vi "Initialize 1553 Module.vi"(4 "Debug Flags (0x3000 0000)":T2, 6 "self test mode (none)":T4(ring), 8 "error in":errorcluster, 10 "BIU number (0)":u8, 11 "module number (0)":u32) -> (0 "error out":errorcluster {"code" format="%x"}, 3 "module reference":T1)   [LabVIEW 2020, in "AIM MIL-STD-1553 Hardware API.lvlib"]
uses:
  AIM MIL-STD-1553 Hardware API.lvlib
  Module Reference.ctl
  <instrlib>/_AIM MIL-STD-1553/PCI-1553 Mid-Level Release/1553 Utility - RT Mode Global.vi
panel:
  out "Reset Information":T3 {"Sim Buffer Addr" format="%08x"; "Sim Buffer Size" format="%08x"; "Bus Mon Buffer Addr" format="%08x"; "Bus Mon Buffer Size" format="%08x"}
  # "Simulator Buffer"
  # "Size"
  # "Address"
  # "Bus Monitor Buffer"
  # "Size"
  # "Address"
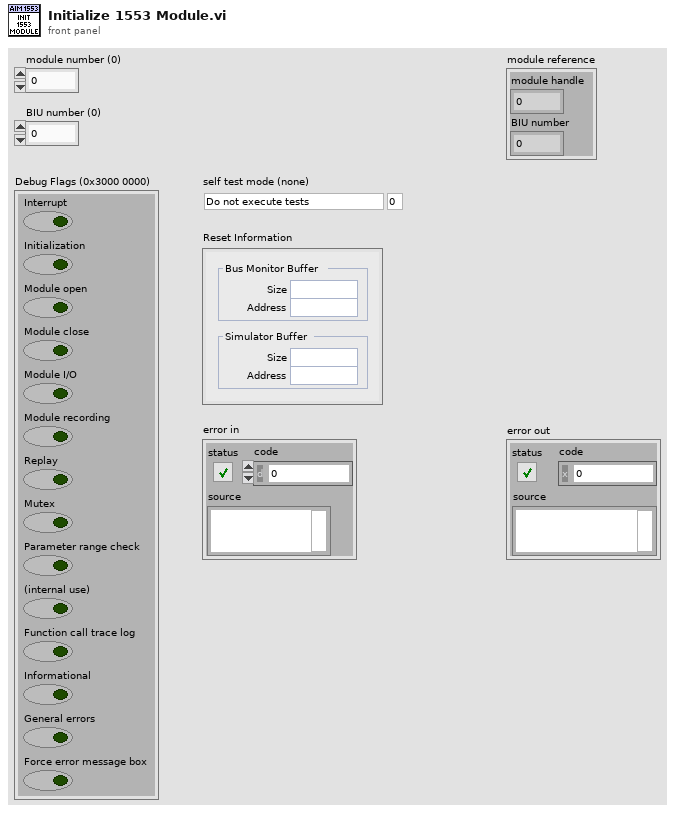
[diagram p1: front panel]
types:
  T1 = typedef "AIM MIL-STD-1553 Hardware API.lvlib/Module Reference.ctl" = cluster{"module handle":u32, "BIU number":u8}
  T2 = cluster{"Interrupt":bool, "Initialization":bool, "Module open":bool, "Module close":bool, "Module I/O":bool, "Module recording":bool, "Replay":bool, "Mutex":bool, "Parameter range check":bool, "(internal use)":bool, "Function call trace log":bool, "Informational":bool, "General errors":bool, "Force error message box":bool}
  T3 = cluster{"Bus Mon Buffer Size":u8, "Sim Buffer Size":u8, "Bus Mon Buffer Addr":u32, "Sim Buffer Addr":u32}
  T4 = enum16{"Do not execute tests", "Execute all tests", "Board enable test", "Internal self-test", "Global RAM test for BIU control block", "Global RAM test for BIU BC/RT descriptor", "Global RAM test for BIU bus monitor", "Shared RAM test from 0x100000", "Shared RAM test for CMD area", "Shared RAM test for ACK area", "Transfer test", "Interrupt test", "DAC test for bus A", "DAC test for bus B", "Timing test"}
  T5 = enum16{"Execute all tests", "Board enable test", "Internal self-test", "Global RAM test for BIU control block", "Global RAM test for BIU BC/RT descriptor", "Global RAM test for BIU bus monitor", "Shared RAM test from 0x100000", "Shared RAM test for CMD area", "Shared RAM test for ACK area", "Transfer test", "Interrupt test", "DAC test for bus A", "DAC test for bus B", "Timing test"}
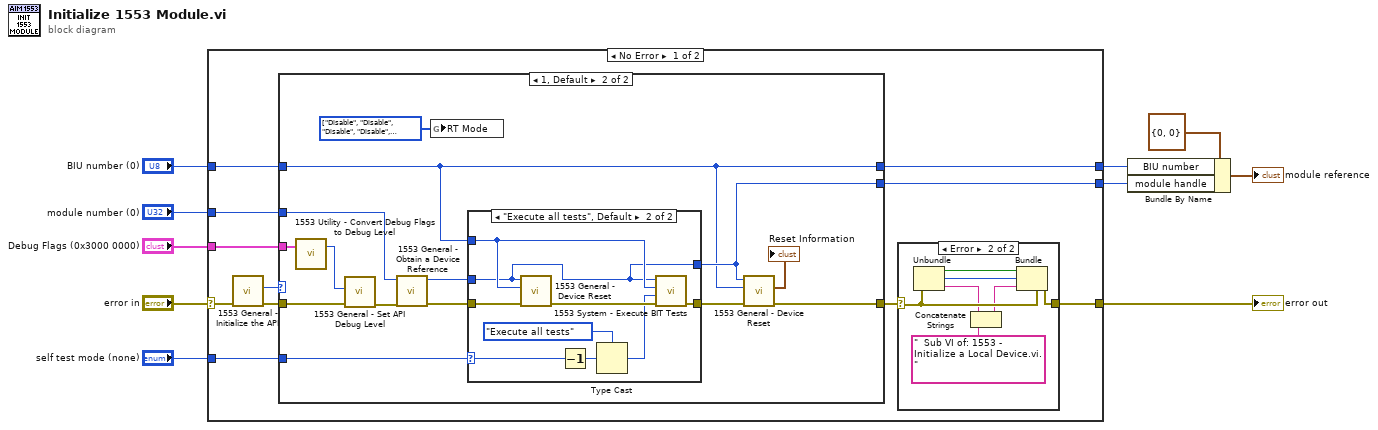
[diagram p0: block diagram]
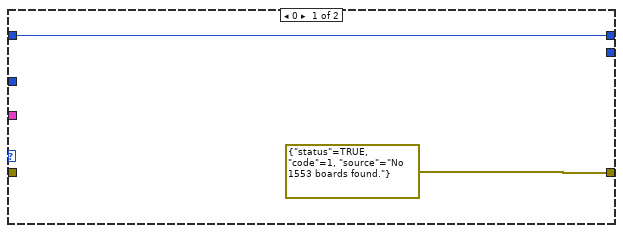
[diagram p3: hidden frame]
diagram:
  n1 = case shown="No Error" "error in" {
    selector: "error in" -> [w18 w58]
    tunnel: [w19 w58] -> w10
    tunnel: [w21 _] -> w3
    tunnel: "module number (0)" -> [w15 _]
    tunnel: "Debug Flags (0x3000 0000)" -> [w14 _]
    tunnel: "self test mode (none)" -> [w13 _]
    tunnel: "BIU number (0)" -> [w12 w57]
    tunnel: [w11 w57] -> w2
    frame No Error {
      n2 = call <instrlib>:"1553 General - Initialize the API.vi"("Error In (none)"=w18) -> ("Error Out"=w17:errorcluster, "Modules Found"=w16:i32)  [unwired: 9 in]
      n3 = case shown="1, Default" w16 {
        tunnel: w17 -> [_ w36]
        tunnel: [errorcluster {"status"=TRUE, "code"=1, "source"="No 1553 boards found."} ("Error Out") w41] -> w20
        tunnel: w14 -> [_ w44]
        tunnel: w13 -> [_ w39]
        tunnel: w15 -> [_ w45]
        tunnel: [_ w34] -> w21
        tunnel: w12 -> [w30 w32]
        tunnel: [w30 w32] -> w11
        frame 0 {
        }
        frame 1, Default {
          w38 = enum16{"Disable", "Simulation", "Monitor"}[] [enum."Disable", enum."Disable", enum."Disable", enum."Disable", enum."Disable", enum."Disable", enum."Disable", enum."Disable", enum."Disable", enum."Disable", enum."Disable", enum."Disable", enum."Disable", enum."Disable", enum."Disable", enum."Disable", enum."Disable", enum."Disable", enum."Disable", enum."Disable", enum."Disable", enum."Disable", enum."Disable", enum."Disable", enum."Disable", enum."Disable", enum."Disable", enum."Disable", enum."Disable", enum."Disable", enum."Disable", enum."Disable"] items=["Disable", "Simulation", "Monitor"] ("RT Mode")
          n4 = call <instrlib>:"1553 Utility - Convert Debug Flags to Debug Level.vi"("Debug Flags (0x3000 0000)"=w44) -> ("Debug Level"=w43:u32)  [unwired: 2 in]
          n5 = call <instrlib>:"1553 General - Set API Debug Level.vi"("Error In (none)"=w36, "Debug Level (0x3000 0000)"=w43) -> ("Error Out"=w35:errorcluster)  [unwired: 9 in]
          n6 = call <instrlib>:"1553 General - Obtain a Device Reference.vi"("Error In (none)"=w35, "Module Number (0)"=w45) -> ("Error Out"=w37:errorcluster, "Module Handle"=w40:u32)  [unwired: 8 in]
          n7 = global write "1553 Utility - RT Mode Global.vi" "RT Mode"(w38) -> ()
          n8 = case shown="\"Execute all tests\", Default" w39 {
            selector: w39 -> [_ w53]
            tunnel: w37 -> [w47 w56]
            tunnel: [w47 w54] -> w42
            tunnel: w40 -> [w46 w48]
            tunnel: w32 -> [_ w49]
            tunnel: [w46 w48] -> w34
            frame "Do not execute tests" {
            }
            frame "Execute all tests", Default {
              n9 = call <instrlib>:"1553 General - Device Reset.vi"("Error In (none)"=w56, "BIU Number (1)"=w49, "Module Handle"=w48) -> ("Error Out"=w55:errorcluster)  [unwired: 7 in, 1 out]
              n10 = Decrement(x=w53) -> (x-1=w52:T4)
              n11 = Type Cast(type=T5."Execute all tests" ("Self test mode (all)"), x=w52) -> (*(type *) &x=w51:T5)
              n12 = call <instrlib>:"1553 System - Execute BIT Tests.vi"("Error In (none)"=w55, "Self test mode (all)"=w51, "BIU Number (1)"=w49, "Module Handle"=w48) -> ("Error Out"=w54:errorcluster)  [unwired: 6 in, 1 out]
            }
          }
          n13 = call <instrlib>:"1553 General - Device Reset.vi"("Error In (none)"=w42, "BIU Number (1)"=w32, "Module Handle"=w34) -> ("Error Out"=w41:errorcluster, "Reset Information"=→"Reset Information":T3)  [unwired: 7 in]
        }
      }
      n14 = case shown="Error" w20 {
        selector: w20 -> [w22 w29]
        tunnel: [w22 w26] -> w19
        frame No Error {
        }
        frame Error {
          n15 = Unbundle(w29) -> ("status"=w27:bool, "code"=w28:i32, "source"=w25:string)
          n16 = Concatenate Strings(w25, "  Sub VI of: 1553 - Initialize a Local Device.vi.") -> (w24:string)
          n17 = Bundle(cluster=w29, "status"=w27, "code"=w28, "source"=w24) -> (w26:errorcluster)
        }
      }
    }
    frame Error {
    }
  }
  "error out" <- w10
  n18 = Bundle By Name(cluster=T1 {"module handle"=0, "BIU number"=0} ("module reference"), "BIU number"=w2, "module handle"=w3) -> (→"module reference":T1)
